vi "Read Spec Page Path.vi"(8 "error in (no error)":errorcluster, 11 "Plugin Generator in":refnum<class "Plugin_Generator.lvclass">) -> (0 "error out":errorcluster, 2 "Path to Spec Page VI":path=path "C:/Program Files/National Instruments/LabVIEW 2021/ProjectTemplates/Source/Delacor/Delacor QMH/scripting/DQMH_SpecPage.vi", 3 "Plugin Generator out":refnum<class "Plugin_Generator.lvclass">)   [LabVIEW 2021, in "Plugin_Generator.lvclass"]
uses:
  Plugin_Generator.lvclass
  Plugin_Generator.lvclass/Plugin_Generator.ctl
panel:
  # "C:\\Program Files\\National Instruments\\LabVIEW 2021\\ProjectTemplates\\Source\\Delacor\\Delacor QMH\\scripting\\DQMH_SpecPage.vi"
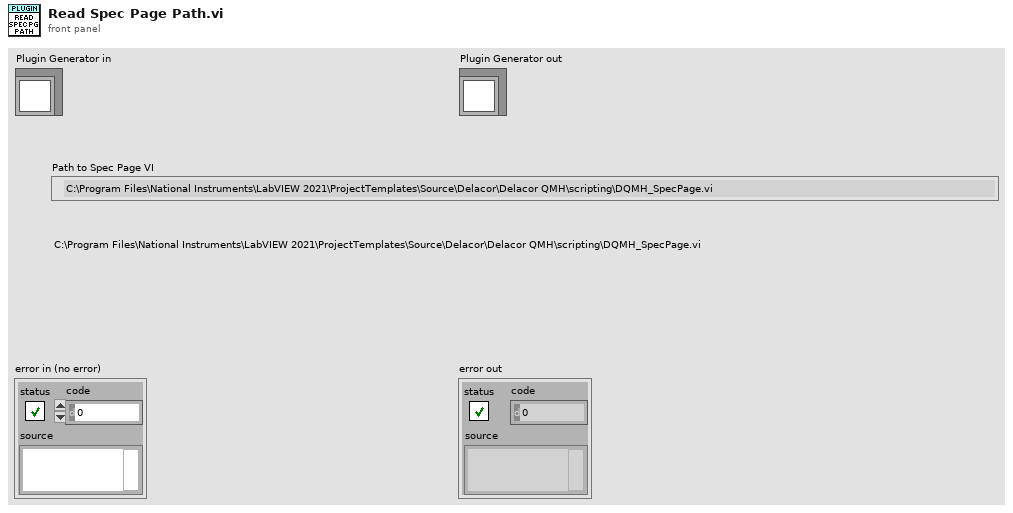
[diagram p1: front panel]
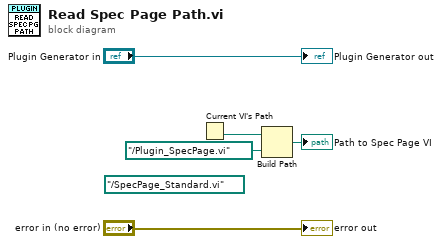
[diagram p0: block diagram]
diagram:
  (unwired) path "../SpecPage_Standard.vi" ("name or relative path")
  n1 = Current VI's Path() -> (path=w3:path)
  n2 = Build Path(base path=w3, name or relative path=path "../Plugin_SpecPage.vi") -> (appended path=→"Path to Spec Page VI":path)
  "error out" <- "error in (no error)"
  "Plugin Generator out" <- "Plugin Generator in"
